vi "Read Avg  values.vi"(8 "error in (no error)":errorcluster, 11 "Temperature Controller Driver in":refnum<class "Temperature Controller Driver.lvclass">) -> (0 "error out":errorcluster, 2 "Avg  values":dbl[](array[numeric]), 3 "Temperature Controller Driver out":refnum<class "Temperature Controller Driver.lvclass">)   [LabVIEW 2024, in "Temperature Controller Driver.lvclass"]
uses:
  Temperature Controller Driver.lvclass
  Temperature Controller Driver.lvclass/Temperature Controller Driver.ctl
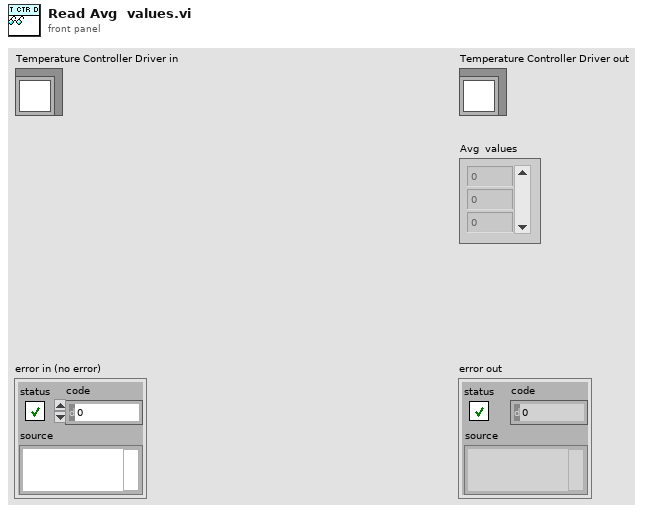
[diagram p1: front panel]
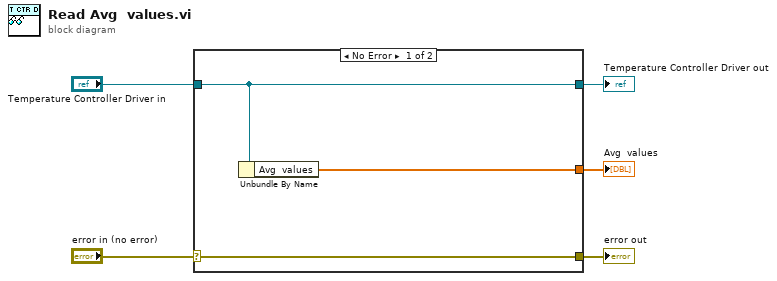
[diagram p0: block diagram]
diagram:
  n1 = case shown="No Error" "error in (no error)" {
    selector: "error in (no error)" -> [w8 w9]
    tunnel: [w8 w9] -> w4
    tunnel: [w7 w10] -> w2
    tunnel: "Temperature Controller Driver in" -> [w7 w10]
    tunnel: [w6 _] -> w1
    frame No Error {
      n2 = Unbundle By Name(w7) -> ("Avg  values"=w6:dbl[])
    }
    frame Error {
    }
  }
  "error out" <- w4
  "Temperature Controller Driver out" <- w2
  "Avg  values" <- w1
